vi "AB_API Set Destination Path.vi"(8 "error in (no error)":errorcluster, 9 "Destination path":path, 10 "Destination label":string, 11 "Build in":refnum<class "AB_Build.lvclass">) -> (0 "error out":errorcluster, 3 "Build out":refnum<class "AB_Build.lvclass">)   [LabVIEW 2020]
uses:
  <vilib>/AppBuilder/AB_Classes/Build/AB_Build.lvclass
  <vilib>/Utility/error.llb/whitespace.ctl
  <vilib>/AppBuilder/AB_Classes/Destination/AB_Destination.lvclass
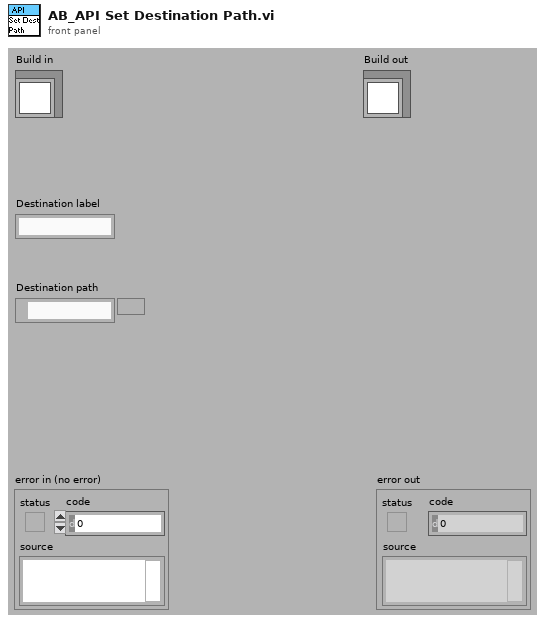
[diagram p1: front panel]
types:
  T1 = typedef "whitespace.ctl" = u16
  T2 = typedef "AB_Build.ctl" = cluster{"buildSpecName":string, "buildSpecDescription":string, "destinations":refnum<class "AB_Destination.lvclass">[], "exclusionOption":T3, "defaultLanguage":string, "supportedLanguages":string[], "excludedDirectories":path[], "buildContext":refnum<vi>, "buildObject":T4, "preview":bool, "programatic":bool, "progressBarEvents":T5, "userLog_Path":path, "preActionID":string, "preAction_Path":path, "postActionID":string, "postAction_Path":path, "eng_checkForBrokenVIs?":bool, "eng_verboseLinkerErrors?":bool, "localDest_Path":path, "targetDest_Path":path, "removeVIObject":u16, "cache":refnum<class "PreviewCache.lvclass">, "use cache":bool, "previewCache_ID":string, "buildCache_ID":string, "eng_TempLocalDest_Path":path, "eng_collectDependencies?":bool, "versionInfo":cluster{"buildVersion":cluster{"major":u16, "minor":u16, "patch":u16, "build":u16}, "autoIncrement":bool}, "eng_enableVIChecksums":bool}
  T3 = typedef "AB_Exclusion_Option.ctl" = cluster{"typedefs":bool, "polymorphicVIs":bool, "unusedLibraryItems":bool, "modifyLibraryFile":bool, "edit-timeDependencies":bool, "inlineVIs":bool, "dependent PPLs":bool, "dependent DLLs":bool}
  T4 = typedef "ItemRef.ctl" = u64
  T5 = typedef "provcom_ProgressBar_Events.ctl" = cluster{"newJob":refnum<user-event>, "newItem":refnum<user-event>, "errorMsg":T6, "cancel":refnum<user-event>}
  T6 = typedef "mxLvBuildError.ctl" = refnum<user-event>
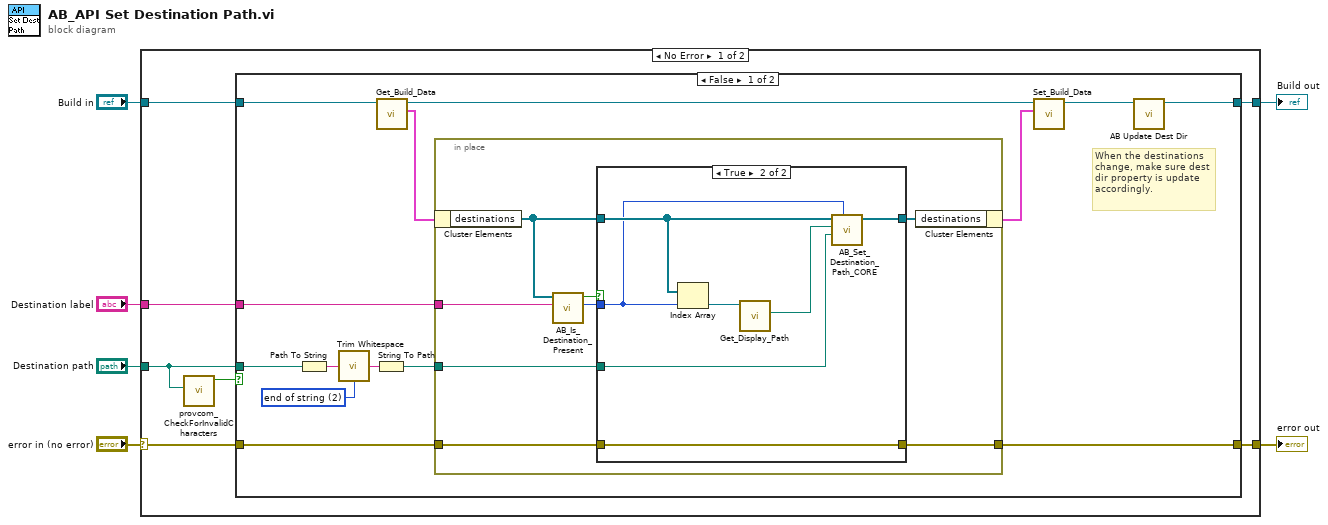
[diagram p0: block diagram]
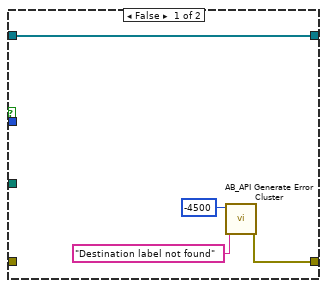
[diagram p2: hidden frame]
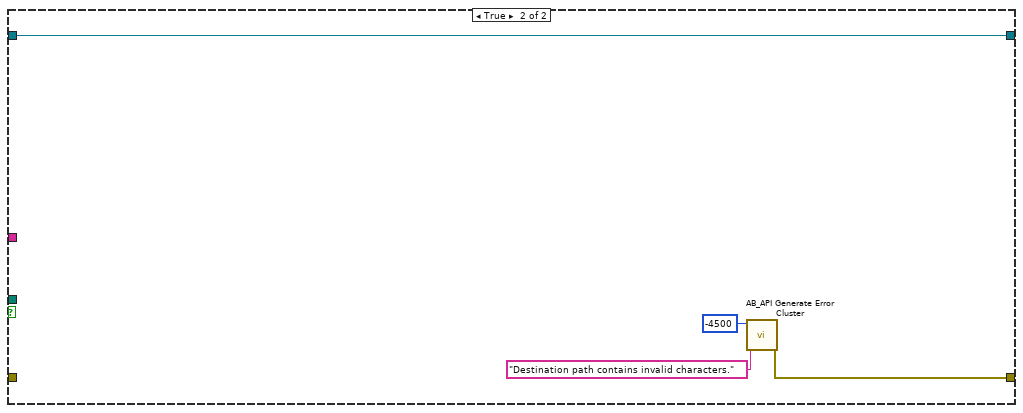
[diagram p3: hidden frame]
diagram:
  n1 = case shown="No Error" "error in (no error)" {
    selector: "error in (no error)" -> [w12 w52]
    tunnel: [w11 w52] -> w5
    tunnel: "Destination label" -> [w13 _]
    tunnel: "Destination path" -> [w8 _]
    tunnel: [w10 w51] -> w2
    tunnel: "Build in" -> [w9 w51]
    frame No Error {
      n2 = call <resource>:"provcom_CheckForInvalidCharacters.vi"("NewPath"=w8) -> ("HasInvalidCharacters"=w7:bool)  [unwired: 2 in, 8 out]
      n3 = case shown="False" w7 {
        tunnel: w13 -> [w24 _]
        tunnel: w12 -> [w23 _]
        tunnel: [w22 w48] -> w11
        tunnel: [w14 w47] -> w10
        tunnel: w9 -> [w21 w47]
        tunnel: w8 -> [w17 _]
        frame False {
          w20 = T1 2 items=["both", "start of string", "end of string"] ("location (both)")
          # "When the destinations change, make sure dest dir property is update accordingly."
          n4 = Path To String(path=w17) -> (string=w18:string)
          n5 = call <vilib>:"Trim Whitespace.vi"("string"=w18, "location (both)"=w20) -> ("trimmed string"=w19:string)
          n6 = String To Path(string=w19) -> (path=w16:path)
          n7 = call <vilib>:"Get_Build_Data.vi"("Class in"=w21) -> ("data"=w26:T2, "Class out"=w27:refnum<class "AB_Build.lvclass">)  [unwired: 1 in, 8 out]
          n8 = in-place {
            in-place-border: w24 -> [w28]
            in-place-border: w16 -> [w34]
            in-place-border: [w32] -> w22
            in-place-border: w23 -> [w31]
            n9 = in-place-cluster #1(w26) -> ("destinations"=w29:refnum<class "AB_Destination.lvclass">[])
            n10 = call <vilib>:"AB_Is_Destination_Present.vi"("destination label"=w28, "destinations"=w29) -> ("index"=w30:i32, "destination present?"=w33:bool)  [unwired: 3 in, 5 out]
            n11 = case shown="True" w33 {
              tunnel: w29 -> [w39 w44]
              tunnel: [w39 w45] -> w35
              tunnel: w30 -> [_ w43]
              tunnel: w34 -> [_ w40]
              tunnel: [w36 w46] -> w32
              tunnel: w31 -> [_ w46]
              frame False {
                n12 = call <vilib>:"AB_API Generate Error Cluster.vi"("Additional Message"="Destination label not found", "Code"=-4500) -> ("error out"=w36:errorcluster)  [unwired: 2 in, 7 out]
              }
              frame True {
                n13 = Index Array(array=w44, index=w43) -> (element=w42:refnum<class "AB_Destination.lvclass">)
                n14 = call-dynamic "Get_Display_Path.vi"("AB_Destination in"=w42) -> ("displayPath"=w41:path)  [unwired: 1 in, 9 out]
                n15 = call <vilib>:"AB_Set_Destination_Path_CORE.vi"("index"=w43, "new path"=w40, "old path"=w41, "destinations in"=w44) -> ("destinations out"=w45:refnum<class "AB_Destination.lvclass">[])  [unwired: 4 in, 3 out]
              }
            }
            n16 = in-place-cluster #1("destinations"=w35) -> (w25:T2)
          }
          n17 = call <vilib>:"Set_Build_Data.vi"("data"=w25, "Class in"=w27) -> ("Class out"=w15:refnum<class "AB_Build.lvclass">)  [unwired: 1 in, 8 out]
          n18 = call <vilib>:"AB Update Dest Dir.vi"("Build in"=w15) -> ("Build out"=w14:refnum<class "AB_Build.lvclass">)  [unwired: 9 in, 1 out]
        }
        frame True {
          n19 = call <vilib>:"AB_API Generate Error Cluster.vi"("Additional Message"="Destination path contains invalid characters.", "Code"=-4500) -> ("error out"=w48:errorcluster)  [unwired: 2 in, 7 out]
        }
      }
    }
    frame Error {
    }
  }
  "error out" <- w5
  "Build out" <- w2
